vi "20TVTI-Merge-Cluster.vi"(1 "VTI Control":T3, 2 "VTI Status":T2={"Temperatur (K)"=70.6986, "Heater (%)"=0.0017142857142857142, "NV (%)"=0.0, "Heater Manual"=TRUE, "NV Manual"=TRUE, "Pressure"=1.0208606, "Dewar Pressure"=1.0500276, "Valid?"=FALSE, "Dewar Heater Manual"=FALSE, "Heater (%) Display"=0.0, "NV (%) Display"=0.0, "Dewar Heater (%)"=18.434412358753207, "D-Heater (%) Display"=18.434412358753207} {"Heater (%)" scale=0.0..100.0; "NV (%)" scale=0.0..100.0; "Dewar Heater (%)" scale=0.0..100.0}) -> (0 "VTI Cluster":T1={"Temperatur (K)"=70.6986, "Setpoint (K)"=0.0, "Rate (K/min)"=3.4572, "Heater (%)"=0.0017142857142857142, "NV (%)"=0.0, "Heater Manual"=TRUE, "NV Manual"=TRUE, "Go to Set"=FALSE, "Pressure"=1.0208606, "Dewar Pressure"=1.0500276, "Heater SP"=0.0, "D-Heater SP"=0.0, "Valid?"=FALSE, "Set Heater SP"=FALSE, "Set NV SP"=FALSE, "Set D-Heater SP"=FALSE, "Dewar Heater Manual"=FALSE, "Heater (%) Display"=0.0, "NV (%) Display"=0.0, "NV Setpoint"=0.0, "Dewar Heater (%)"=18.434412358753207, "D-Heater (%) Display"=18.434412358753207, "Change Heater Status"=FALSE, "Change NV Status"=FALSE, "Change D-Heater Status"=FALSE, "Change Sweep Type"=FALSE} {"D-Heater (%) Display" format="%4_5f"; "Dewar Heater (%)" scale=0.0..100.0; "NV (%) Display" format="%4_5f"; "Heater (%) Display" format="%4_5f"; "Dewar Pressure" format="%#4_5f"; "Pressure" format="%#4_5f"; "NV (%)" scale=0.0..100.0; "Heater (%)" scale=0.0..100.0; "Rate (K/min)" format="%#4_5f"; "Setpoint (K)" format="%6_5f"})   [LabVIEW 2016]
uses:
  C:/Users/sweet16/Desktop/Control 1.ctl
  20TVTI_Status.ctl
  20TVTI_Cluster.ctl
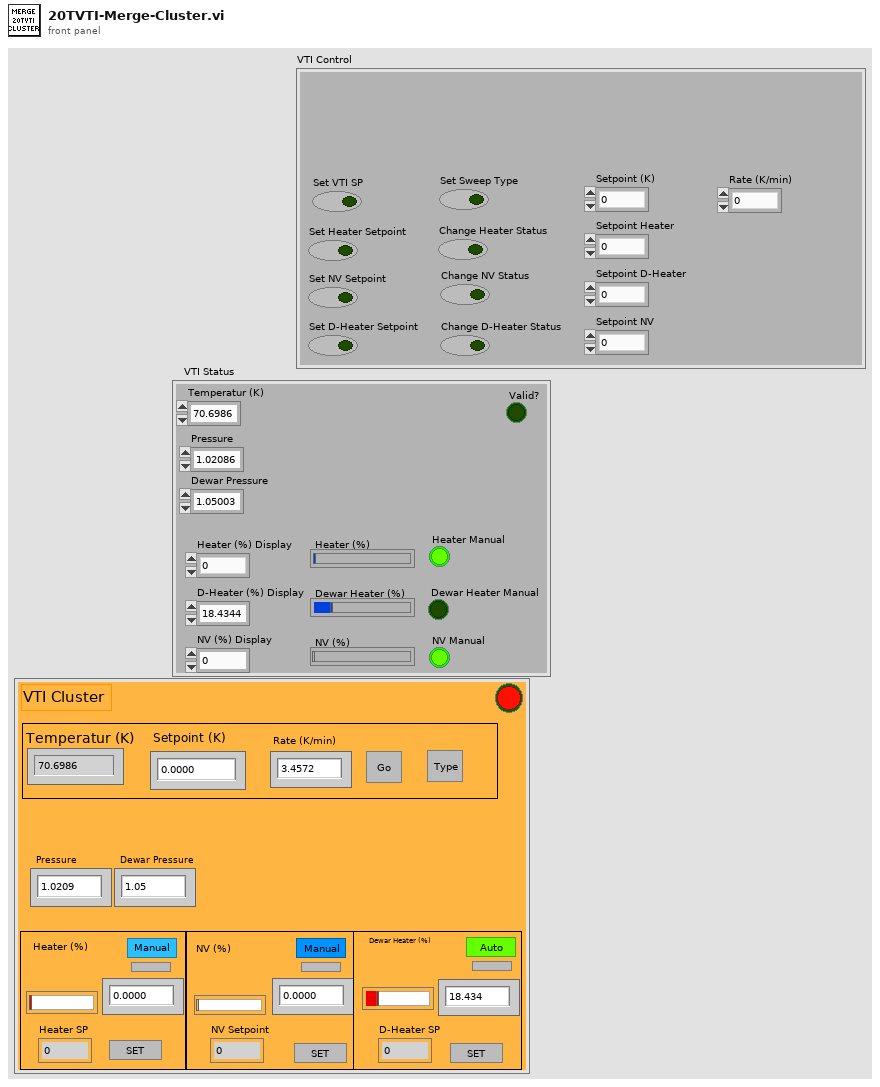
[diagram p1: front panel]
types:
  T1 = typedef "20TVTI_Cluster.ctl" = cluster{"Temperatur (K)":dbl, "Setpoint (K)":dbl, "Rate (K/min)":dbl, "Heater (%)":dbl, "NV (%)":dbl, "Heater Manual":bool, "NV Manual":bool, "Go to Set":bool, "Pressure":dbl, "Dewar Pressure":dbl, "Heater SP":dbl, "D-Heater SP":dbl, "Valid?":bool, "Set Heater SP":bool, "Set NV SP":bool, "Set D-Heater SP":bool, "Dewar Heater Manual":bool, "Heater (%) Display":dbl, "NV (%) Display":dbl, "NV Setpoint":dbl, "Dewar Heater (%)":dbl, "D-Heater (%) Display":dbl, "Change Heater Status":bool, "Change NV Status":bool, "Change D-Heater Status":bool, "Change Sweep Type":bool}
  T2 = typedef "20TVTI_Status.ctl" = cluster{"Temperatur (K)":dbl, "Heater (%)":dbl, "NV (%)":dbl, "Heater Manual":bool, "NV Manual":bool, "Pressure":dbl, "Dewar Pressure":dbl, "Valid?":bool, "Dewar Heater Manual":bool, "Heater (%) Display":dbl, "NV (%) Display":dbl, "Dewar Heater (%)":dbl, "D-Heater (%) Display":dbl}
  T3 = typedef "Control 1.ctl" = cluster{"Set VTI SP":bool, "Change NV Status":bool, "Set NV Setpoint":bool, "Change Heater Status":bool, "Set D-Heater Setpoint":bool, "Set Heater Setpoint":bool, "Change D-Heater Status":bool, "Set Sweep Type":bool, "Setpoint (K)":dbl, "Rate (K/min)":dbl, "Setpoint Heater":dbl, "Setpoint D-Heater":dbl, "Setpoint NV":dbl}
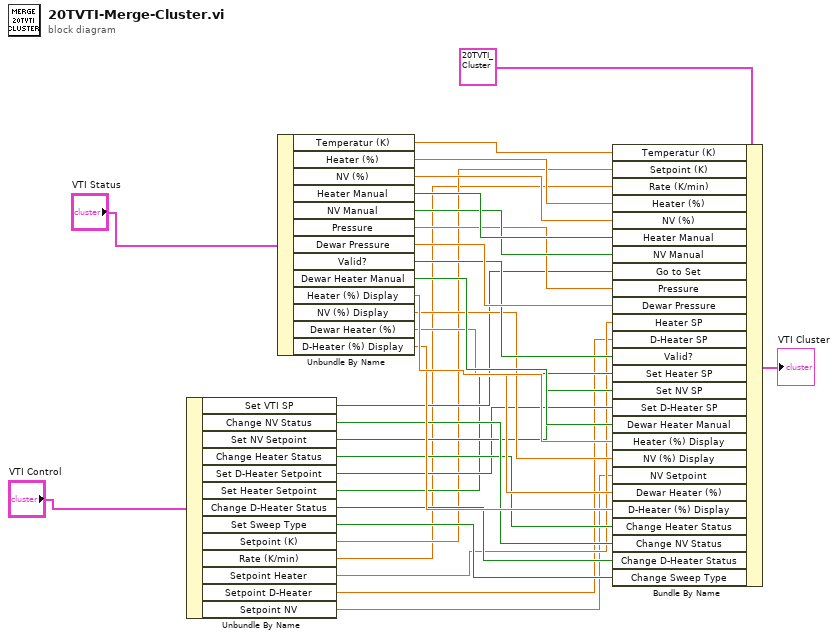
[diagram p0: block diagram]
diagram:
  n1 = Unbundle By Name("VTI Control") -> ("Set VTI SP"=w14:bool, "Change NV Status"=w13:bool, "Set NV Setpoint"=w12:bool, "Change Heater Status"=w11:bool, "Set D-Heater Setpoint"=w10:bool, "Set Heater Setpoint"=w9:bool, "Change D-Heater Status"=w8:bool, "Set Sweep Type"=w7:bool, "Setpoint (K)"=w6:dbl, "Rate (K/min)"=w5:dbl, "Setpoint Heater"=w4:dbl, "Setpoint D-Heater"=w3:dbl, "Setpoint NV"=w2:dbl)
  n2 = Unbundle By Name("VTI Status") -> ("Temperatur (K)"=w27:dbl, "Heater (%)"=w26:dbl, "NV (%)"=w25:dbl, "Heater Manual"=w24:bool, "NV Manual"=w23:bool, "Pressure"=w22:dbl, "Dewar Pressure"=w21:dbl, "Valid?"=w20:bool, "Dewar Heater Manual"=w19:bool, "Heater (%) Display"=w18:dbl, "NV (%) Display"=w17:dbl, "Dewar Heater (%)"=w16:dbl, "D-Heater (%) Display"=w15:dbl)
  n3 = Bundle By Name(cluster=T1 {"Temperatur (K)"=70.6986, "Setpoint (K)"=0.0, "Rate (K/min)"=3.4572, "Heater (%)"=0.0017142857142857142, "NV (%)"=0.0, "Heater Manual"=TRUE, "NV Manual"=TRUE, "Go to Set"=FALSE, "Pressure"=1.0208606, "Dewar Pressure"=1.0500276, "Heater SP"=0.0, "D-Heater SP"=0.0, "Valid?"=FALSE, "Set Heater SP"=FALSE, "Set NV SP"=FALSE, "Set D-Heater SP"=FALSE, "Dewar Heater Manual"=FALSE, "Heater (%) Display"=0.0, "NV (%) Display"=0.0, "NV Setpoint"=0.0, "Dewar Heater (%)"=18.434412358753207, "D-Heater (%) Display"=18.434412358753207, "Change Heater Status"=FALSE, "Change NV Status"=FALSE, "Change D-Heater Status"=FALSE, "Change Sweep Type"=FALSE} ("VTI Cluster 2"), "Temperatur (K)"=w27, "Setpoint (K)"=w6, "Rate (K/min)"=w5, "Heater (%)"=w26, "NV (%)"=w25, "Heater Manual"=w24, "NV Manual"=w23, "Go to Set"=w14, "Pressure"=w22, "Dewar Pressure"=w21, "Heater SP"=w4, "D-Heater SP"=w3, "Valid?"=w20, "Set Heater SP"=w9, "Set NV SP"=w12, "Set D-Heater SP"=w10, "Dewar Heater Manual"=w19, "Heater (%) Display"=w18, "NV (%) Display"=w17, "NV Setpoint"=w2, "Dewar Heater (%)"=w16, "D-Heater (%) Display"=w15, "Change Heater Status"=w11, "Change NV Status"=w13, "Change D-Heater Status"=w8, "Change Sweep Type"=w7) -> (→"VTI Cluster":T1)
